vi "DecideWhenToShift.vi"(4 "Force to Low Gear":bool, 6 "Force To High Gear":bool, 7 "Drive Motor Speed (rpm)":dbl, 8 "Time Below Speed (ms)":u32, 9 "Time Above Speed (ms)":u32, 10 "Switch to Low Gear (rpm)":dbl, 11 "Switch to High Gear (rpm)":dbl) -> (3 "Requested Shifter State":bool)   [LabVIEW 2019]
doc: "This VI decides when to shift a swerve module based on the drive motor RPM. Includes a hysteresis to prevent vacillation."
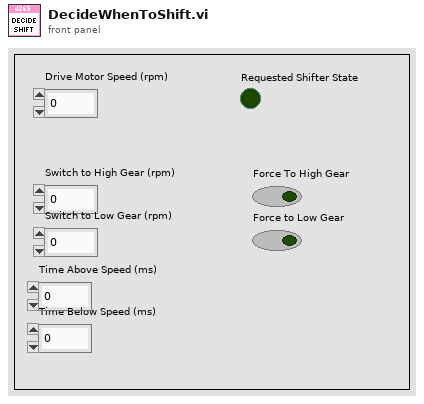
[diagram p1: front panel]
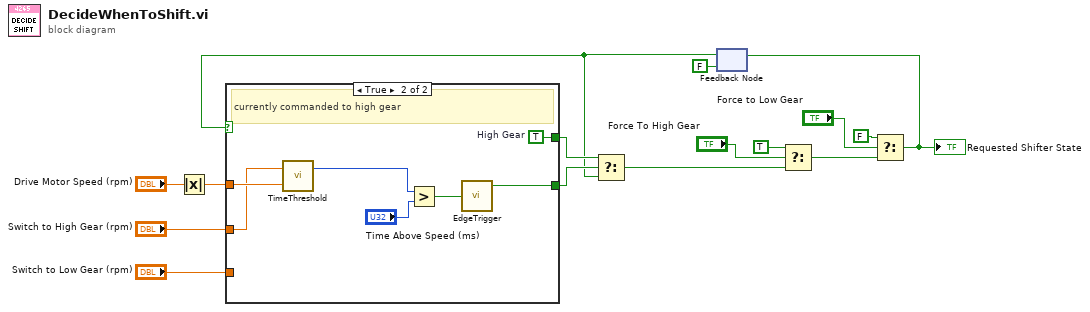
[diagram p0: block diagram]
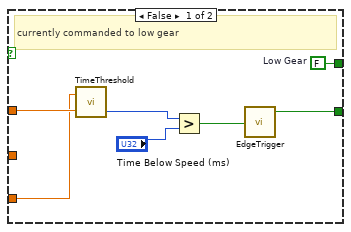
[diagram p2: hidden frame]
diagram:
  n1 = Absolute Value(x="Drive Motor Speed (rpm)") -> (abs(x)=w1:dbl)
  n2 = feedback #1(FALSE ("High Gear")) -> (w2:bool)
  n3 = case shown="True" w2 {
    tunnel: w1 -> [w22 w29]
    tunnel: "Switch to High Gear (rpm)" -> [_ w28]
    tunnel: "Switch to Low Gear (rpm)" -> [w21 _]
    tunnel: [w16 w24] -> w12
    tunnel: [w18 w23] -> w11
    frame False {
      w18 = FALSE  # Low Gear
      # "currently commanded to low gear"
      n4 = call "TimeThreshold.vi"("Threshold"=w22, "Current Value"=w21) -> ("Time Below Threshold (ms)"=w20:u32)  [unwired: 1 out]
      n5 = Greater?(x=w20, y="Time Below Speed (ms)") -> (0:w17:bool)
      n6 = call "EdgeTrigger.vi"("Input Signal"=w17) -> ("Rising Edge Trigger"=w16:bool)  [unwired: 2 out]
    }
    frame True {
      w23 = TRUE  # High Gear
      # "currently commanded to high gear"
      n7 = call "TimeThreshold.vi"("Threshold"=w29, "Current Value"=w28) -> ("Time Above Threshold (ms)"=w27:u32)  [unwired: 1 out]
      n8 = Greater?(x=w27, y="Time Above Speed (ms)") -> (0:w25:bool)
      n9 = call "EdgeTrigger.vi"("Input Signal"=w25) -> ("Rising Edge Trigger"=w24:bool)  [unwired: 2 out]
    }
  }
  n10 = Select(t=w11, s=w12, f=w2) -> (s? t:f=w9:bool)
  n11 = Select(t=TRUE, s="Force To High Gear", f=w9) -> (s? t:f=w8:bool)
  n12 = Select(t=FALSE, s="Force to Low Gear", f=w8) -> (s? t:f=w3:bool)
  "Requested Shifter State" <- w3
  n13 = feedback-in #1(w3) -> ()
